vi "test_ServiceLocationPool_GetLocation_ReturnsValidLocation.vi"(8 "error in (no error)":errorcluster) -> (0 "error out":errorcluster, 2 "result":string, 3 "pass":bool)   [LabVIEW 2020, in "MeasurementServerTests.lvlib"]
uses:
  MeasurementServerTests.lvlib
  Runtime/MeasurementLink Discovery/MeasurementLink Discovery.lvlib
  Runtime/MeasurementLink Discovery Client/RPC Messages/ni_measurementlink_discovery_v1_ResolveServiceRequest.ctl
  Runtime/MeasurementLink Discovery Client/MeasurementLink Discovery Client.lvlib
  Runtime/MeasurementLink Discovery/Service Location FGV Action.ctl
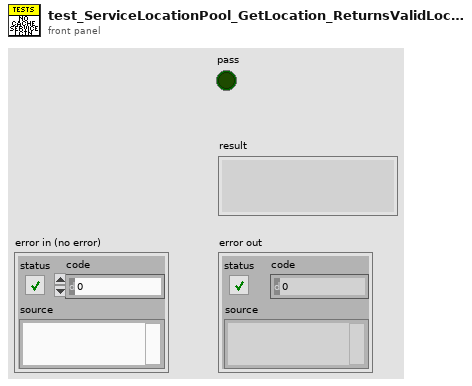
[diagram p1: front panel]
types:
  T1 = typedef "MeasurementLink Discovery Client.lvlib/ni_measurementlink_discovery_v1_ResolveServiceRequest.ctl" = cluster{"provided_interface":string, "service_class":string}
  T2 = typedef "MeasurementLink Discovery.lvlib/Service Location FGV Action.ctl" = enum16{"Get Service Location", "Reresolve Service Location"}
  T3 = typedef "MeasurementLink Discovery Client.lvlib/ni_measurementlink_discovery_v1_ServiceLocation.ctl" = cluster{"location":string, "insecure_port":string, "ssl_authenticated_port":string}
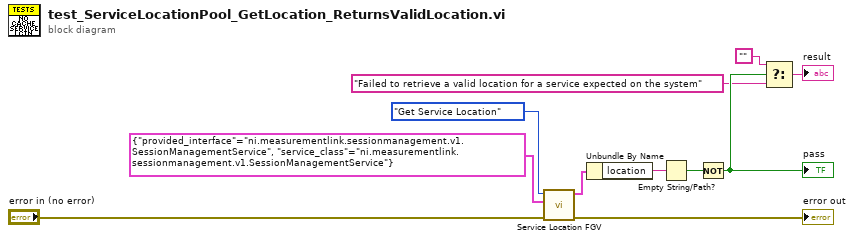
[diagram p0: block diagram]
diagram:
  n1 = call "Service Location FGV.vi"("error in"="error in (no error)", "resolve service request"=T1 {"provided_interface"="ni.measurementlink.sessionmanagement.v1.SessionManagementService", "service_class"="ni.measurementlink.sessionmanagement.v1.SessionManagementService"} ("Resolve Service Request"), "action"=Service_Location_FGV_Action."Get Service Location" ("Action")) -> ("error out"=→"error out":errorcluster, "service location"=w7:T3)  [unwired: 6 in, 1 out]
  n2 = Unbundle By Name(w7) -> ("location"=w6:string)
  n3 = Empty String/Path?(string/path=w6) -> (empty?=w5:bool)
  n4 = Not(x=w5) -> (.not. x?=w3:bool)
  "pass" <- w3
  n5 = Select(t="", s=w3, f="Failed to retrieve a valid location for a service expected on the system") -> (s? t:f=→"result":string)
